vi "PointInPolygon.vi"(1 "Polygon":T1, 2 "2DPoint":T2) -> (0 "InPolygon":bool)   [LabVIEW 2017]
uses:
  TypeDefs/Point2D.ctl
  TypeDefs/Polygon2D.ctl
  <vilib>/Analysis/geometry.llb/Point in Polygon Position.ctl
  <vilib>/Analysis/geometry.llb/Point in Polygon (Scalar).vi
  <vilib>/Analysis/NI_AAL_Geometry.lvlib
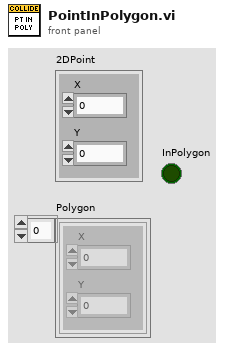
[diagram p1: front panel]
types:
  T1 = typedef "Polygon2D.ctl" = T2[]
  T2 = typedef "Point2D.ctl" = cluster{"X":dbl, "Y":dbl}
  T3 = typedef "NI_AAL_Geometry.lvlib/Point in Polygon Position.ctl" = u16
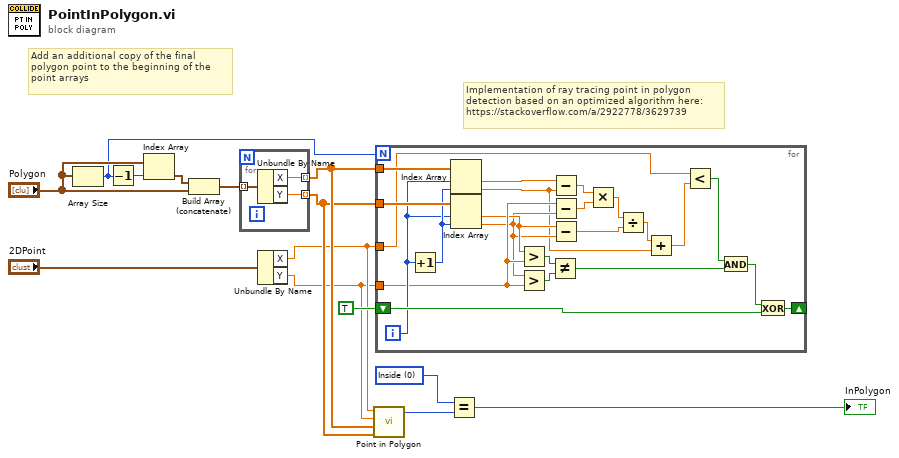
[diagram p0: block diagram]
diagram:
  w6 = T3 0 items=["Inside", "On Boundary", "Outside"] ("x")
  # "Add an additional copy of the final\npolygon point to the beginning of the\npoint arrays"
  # "Implementation of ray tracing point in polygon\ndetection based on an optimized algorithm here:\nhttps://stackoverflow.com/a/2922778/3629739"
  n1 = Array Size(array="Polygon") -> (size(s)=w8:i32)
  n2 = Decrement(x=w8) -> (x-1=w11:i32)
  n3 = Index Array(array="Polygon", index=w11) -> (element=w9:T2)
  n4 = Build Array (concatenate)(w9, "Polygon") -> (w10:T1)
  n5 = for {
    tunnel: w10 -> [w17] mode=indexing
    tunnel: [w16] -> w4 mode=indexing
    tunnel: [w15] -> w3 mode=indexing
    n6 = Unbundle By Name(w17) -> ("X"=w16:dbl, "Y"=w15:dbl)
  }
  n7 = Unbundle By Name("2DPoint") -> ("X"=w2:dbl, "Y"=w1:dbl)
  n8 = call-poly <vilib>:"Point in Polygon.vi"("Polygon Y"=w3, "Polygon X"=w4, "y"=w1, "x"=w2) -> ("position"=w7:T3)  [unwired: 6 in, 1 out]
  n9 = for {
    N: w8 -> [_]
    shift-right: [w40] -> _
    shift-left: TRUE -> [w39]
    tunnel: w4 -> [w38]
    tunnel: w3 -> [w37]
    tunnel: w2 -> [w30]
    tunnel: w1 -> [w27]
    i -> [w35]
    n10 = Increment(x=w35) -> (x+1=w36:i32)
    n11 = Index Array(array=w38, index #1=w35, index #2=w36) -> (element #1=w28:dbl, element #2=w19:dbl)
    n12 = Index Array(array=w37, index #1=w35, index #2=w36) -> (element #1=w26:dbl, element #2=w25:dbl)
    n13 = Greater?(x=w26, y=w27) -> (0:w33:bool)
    n14 = Greater?(x=w25, y=w27) -> (0:w34:bool)
    n15 = Not Equal?(x=w33, y=w34) -> (x != y?=w32:bool)
    n16 = Subtract(x=w28, y=w19) -> (x-y=w24:dbl)
    n17 = Subtract(x=w27, y=w25) -> (x-y=w23:dbl)
    n18 = Subtract(x=w26, y=w25) -> (x-y=w21:dbl)
    n19 = Multiply(x=w24, y=w23) -> (x*y=w22:dbl)
    n20 = Divide(x=w22, y=w21) -> (x/y=w20:dbl)
    n21 = Add(x=w20, y=w19) -> (x+y=w18:dbl)
    n22 = Less?(x=w30, y=w18) -> (x < y?=w29:bool)
    n23 = And(x=w29, y=w32) -> (x .and. y?=w31:bool)
    n24 = Exclusive Or(1:w39, 2:w31) -> (0:w40:bool)
  }
  n25 = Equal?(x=w6, y=w7) -> (x = y?=→"InPolygon":bool)
